vi "CIPC Post-Install Custom Action.vi"(10 "Variant":variant) -> (0 "error out":errorcluster)   [LabVIEW 2021]
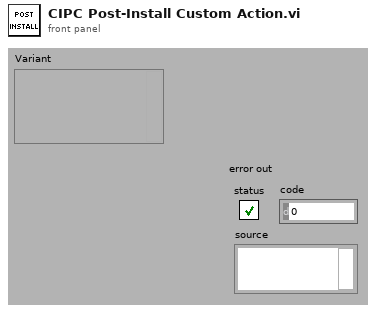
[diagram p1: front panel]
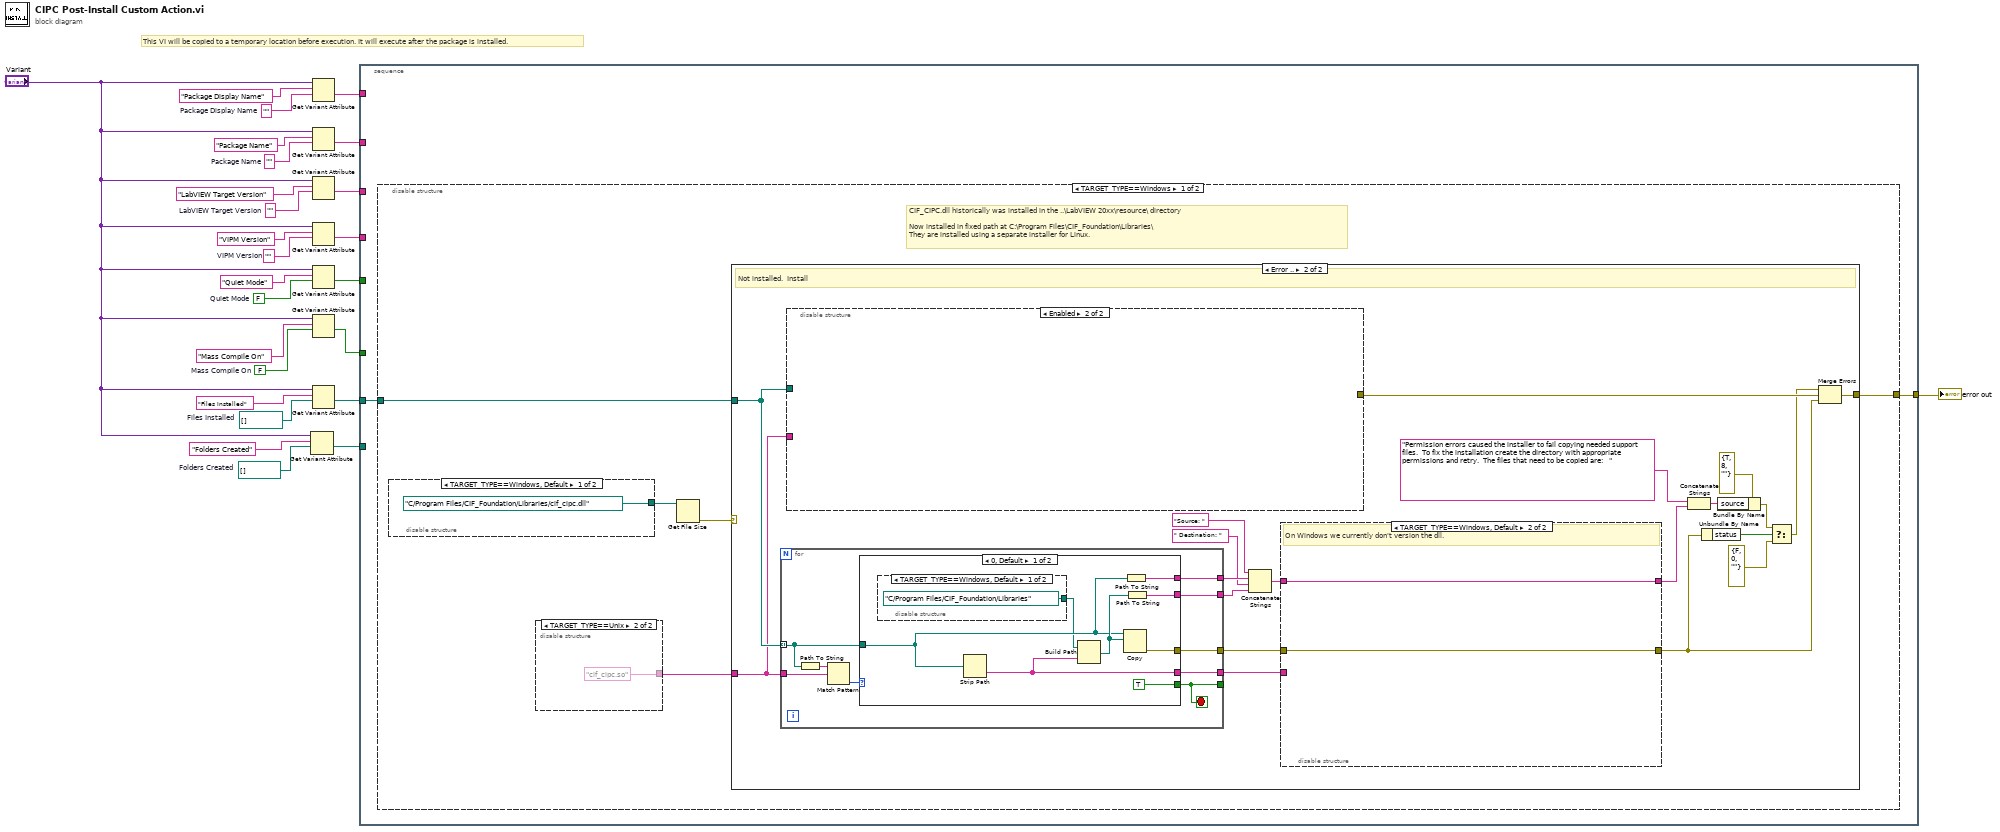
[diagram p0: block diagram]
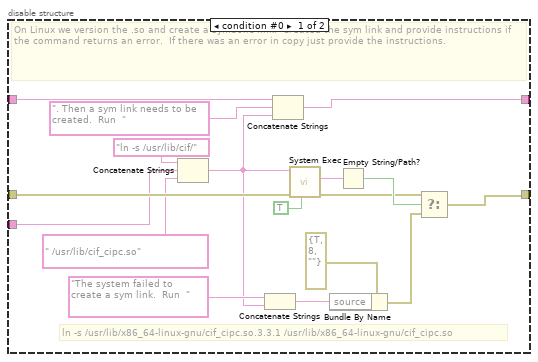
[diagram p3: hidden frame]
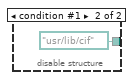
[diagram p4: hidden frame]
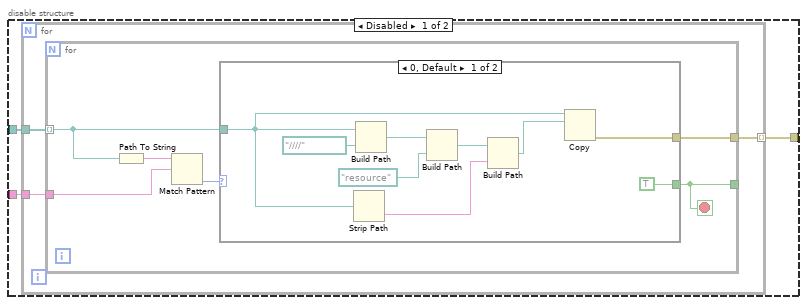
[diagram p6: hidden frame]
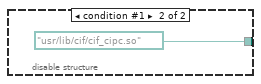
[diagram p8: hidden frame]
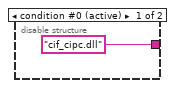
[diagram p9: hidden frame]
diagram:
  w2 = path[] []  # Folders Created
  w3 = path[] []  # Files Installed
  w9 = FALSE  # Mass Compile On
  w10 = ""  # Package Display Name
  w17 = FALSE  # Quiet Mode
  w20 = ""  # VIPM Version
  w22 = ""  # LabVIEW Target Version
  w24 = ""  # Package Name
  # "This VI will be copied to a temporary location before execution. It will execute after the package is installed."
  n1 = Get Variant Attribute(Variant="Variant", name="Folders Created", default value (empty Variant)=w2) -> (value=w7:path[])  [unwired: 1 in, 3 out]
  n2 = Get Variant Attribute(Variant="Variant", name="Package Display Name", default value (empty Variant)=w10) -> (value=w16:string)  [unwired: 1 in, 3 out]
  n3 = Get Variant Attribute(Variant="Variant", name="Package Name", default value (empty Variant)=w24) -> (value=w15:string)  [unwired: 1 in, 3 out]
  n4 = Get Variant Attribute(Variant="Variant", name="LabVIEW Target Version", default value (empty Variant)=w22) -> (value=w14:string)  [unwired: 1 in, 3 out]
  n5 = Get Variant Attribute(Variant="Variant", name="VIPM Version", default value (empty Variant)=w20) -> (value=w13:string)  [unwired: 1 in, 3 out]
  n6 = Get Variant Attribute(Variant="Variant", name="Quiet Mode", default value (empty Variant)=w17) -> (value=w12:bool)  [unwired: 1 in, 3 out]
  n7 = Get Variant Attribute(Variant="Variant", name="Mass Compile On", default value (empty Variant)=w9) -> (value=w11:bool)  [unwired: 1 in, 3 out]
  n8 = Get Variant Attribute(Variant="Variant", name="Files Installed", default value (empty Variant)=w3) -> (value=w6:path[])  [unwired: 1 in, 3 out]
  n9 = stacked-sequence {
    tunnel: w16 -> [_]
    tunnel: w15 -> [_]
    tunnel: w14 -> [_]
    tunnel: w13 -> [_]
    tunnel: w12 -> [_]
    tunnel: w11 -> [_]
    tunnel: w6 -> [w27]
    tunnel: w7 -> [_]
    tunnel: [w28] -> w1
    frame #0 {
      n10 = disable-structure shown="TARGET_TYPE==Windows" {
        disable-tunnel: [w33 _] -> w28
        disable-tunnel: w27 -> [w32 _]
        frame condition #0 (active) {
          # "CIF_CIPC.dll historically was installed in the ..\\LabVIEW 20xx\\resource\\ directory\n\nNow installed in fixed path at C:\\Program Files\\CIF_Foundation\\Libraries\\ \nThey are installed using a separate installer for Linux."
          n11 = disable-structure shown="TARGET_TYPE==Windows, Default" {
            disable-tunnel: [path "C:/Program Files/CIF_Foundation/Libraries/cif_cipc.dll" ("Path In") path "/usr/lib/cif/cif_cipc.so" ("Path In")] -> w30
            frame condition #0 (active) {
            }
            frame condition #1 {
            }
          }
          n12 = disable-structure shown="TARGET_TYPE==Unix" {
            disable-tunnel: ["cif_cipc.dll" ("regular expression") "cif_cipc.so" ("regular expression")] -> w31
            frame condition #0 (active) {
            }
            frame condition #1 {
            }
          }
          n13 = Get File Size(file=w30) -> (0:w29:errorcluster)  [unwired: 1 in, 2 out]
          n14 = case shown="Error .." w29 {
            tunnel: [_ w52] -> w33
            tunnel: w32 -> [_ w51]
            tunnel: w31 -> [_ w46]
            frame No Error {
              # "Already installed.  Skip installation step.  This is needed because we removed the uninstall step from VIPM."
            }
            frame Error {
              # "Not installed.  Install"
              n15 = for {
                tunnel: w51 -> [w79] mode=indexing
                tunnel: [w78] -> _
                tunnel: w46 -> [w77]
                tunnel: [w76] -> w42
                tunnel: [w75] -> w45
                tunnel: [w74] -> w41
                tunnel: [w73] -> w39
                stop <- w78 stop-if-true
                n16 = Path To String(path=w79) -> (string=w81:string)
                n17 = Match Pattern(string=w81, regular expression=w77) -> (offset past match=w80:i32)  [unwired: 1 in, 3 out]
                n18 = case shown="0, Default" w80 {
                  tunnel: w79 -> [w86 _]
                  tunnel: [TRUE _] -> w78
                  tunnel: [w88 _] -> w76
                  tunnel: [w85 _] -> w75
                  tunnel: [w84 _] -> w74
                  tunnel: [w82 _] -> w73
                  frame 0, Default {
                    n19 = disable-structure shown="TARGET_TYPE==Windows, Default" {
                      disable-tunnel: [path "C:/Program Files/CIF_Foundation/Libraries" ("Path In") path "/usr/lib/cif" ("Path In")] -> w83
                      frame condition #0 (active) {
                      }
                      frame condition #1 {
                      }
                    }
                    n20 = Strip Path(path=w86) -> (name=w82:string)  [unwired: 1 out]
                    n21 = Build Path(base path=w83, name or relative path=w82) -> (appended path=w87:path)
                    n22 = Copy(10:w87, 11:w86) -> (0:w88:errorcluster)  [unwired: 3 in, 2 out]
                    n23 = Path To String(path=w86) -> (string=w85:string)
                    n24 = Path To String(path=w87) -> (string=w84:string)
                  }
                  frame -1 {
                  }
                }
              }
              n25 = disable-structure shown="Enabled" {
                disable-tunnel: [w94 _] -> w53
                disable-tunnel: w46 -> [w93 _]
                disable-tunnel: w51 -> [w92 _]
                frame Disabled {
                  n26 = for {
                    tunnel: w92 -> [w97]
                    tunnel: w93 -> [w96]
                    tunnel: [w95] -> w94 mode=indexing
                    n27 = for {
                      tunnel: w97 -> [w101] mode=indexing
                      tunnel: [w100] -> _
                      tunnel: w96 -> [w99]
                      tunnel: [w98] -> w95
                      stop <- w100 stop-if-true
                      n28 = Path To String(path=w101) -> (string=w103:string)
                      n29 = Match Pattern(string=w103, regular expression=w99) -> (offset past match=w102:i32)  [unwired: 1 in, 3 out]
                      n30 = case shown="0, Default" w102 {
                        tunnel: w101 -> [w105 _]
                        tunnel: [TRUE _] -> w100
                        tunnel: [w104 _] -> w98
                        frame 0, Default {
                          n31 = Strip Path(path=w105) -> (name=w108:string)  [unwired: 1 out]
                          n32 = Build Path(base path=w105, name or relative path=path "../../../../..") -> (appended path=w111:path)
                          n33 = Build Path(base path=w111, name or relative path=path "resource") -> (appended path=w109:path)
                          n34 = Build Path(base path=w109, name or relative path=w108) -> (appended path=w106:path)
                          n35 = Copy(10:w106, 11:w105) -> (0:w104:errorcluster)  [unwired: 3 in, 2 out]
                        }
                        frame -1 {
                        }
                      }
                    }
                  }
                }
                frame Enabled {
                }
              }
              n36 = Concatenate Strings("Source: " ("string"), w45, " Destination: " ("string"), w41) -> (w40:string)
              n37 = disable-structure shown="TARGET_TYPE==Windows, Default" {
                disable-tunnel: w42 -> [w70 w72]
                disable-tunnel: [w55 w72] -> w36
                disable-tunnel: w40 -> [w66 w71]
                disable-tunnel: w39 -> [w61 _]
                disable-tunnel: [w56 w71] -> w38
                frame condition #0 {
                  # "ln -s /usr/lib/x86_64-linux-gnu/cif_cipc.so.3.3.1 /usr/lib/x86_64-linux-gnu/cif_cipc.so"
                  # "On Linux we version the .so and create a symbolic link.  Created the sym link and provide instructions if the command returns an error.  If there was an error in copy just provide the instructions."
                  n38 = Concatenate Strings("ln -s /usr/lib/cif/" ("string"), w61, " /usr/lib/cif_cipc.so" ("string")) -> (w60:string)
                  n39 = Concatenate Strings("The system failed to create a sym link.  Run  " ("string"), w60) -> (w65:string)
                  n40 = Concatenate Strings(w66, ". Then a sym link needs to be created.  Run  " ("string"), w60) -> (w56:string)
                  n41 = call <vilib>:"System Exec.vi"("run minimized? (F)"=TRUE, "error in (no error)"=w70, "command line"=w60) -> ("error out"=w54:errorcluster, "standard error"=w68:string)  [unwired: 5 in, 2 out]
                  n42 = Bundle By Name(cluster=errorcluster {"status"=TRUE, "code"=8, "source"=""} ("t"), "source"=w65) -> (w62:errorcluster)
                  n43 = Empty String/Path?(string/path=w68) -> (empty?=w67:bool)
                  n44 = Select(t=w54, s=w67, f=w62) -> (s? t:f=w55:errorcluster)
                }
                frame condition #1 (active) {
                  # "On Windows we currently don't version the dll."
                }
              }
              n45 = Concatenate Strings("Permission errors caused the installer to fail copying needed support files.  To fix the installation create the directory with appropriate permissions and retry.  The files that need to be copied are:   " ("string"), w38) -> (w47:string)
              n46 = Unbundle By Name(w36) -> ("status"=w37:bool)
              n47 = Bundle By Name(cluster=errorcluster {"status"=TRUE, "code"=8, "source"=""} ("t"), "source"=w47) -> (w48:errorcluster)
              n48 = Select(t=w48, s=w37, f=errorcluster {"status"=FALSE, "code"=0, "source"=""}) -> (s? t:f=w50:errorcluster)
              n49 = Merge Errors(w50, w53, w36) -> (w52:errorcluster)
            }
          }
        }
        frame condition #1 {
        }
      }
    }
  }
  "error out" <- w1
